vi "bmp_2_file(processed).vi"(10 "Dest":path, 11 "Image":path) -> ()   [LabVIEW 2015]
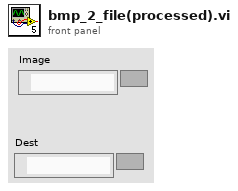
[diagram p1: front panel]
types:
  T1 = enum16{"open", "replace", "create", "open or create", "replace or create", "replace or create with confirmation"}
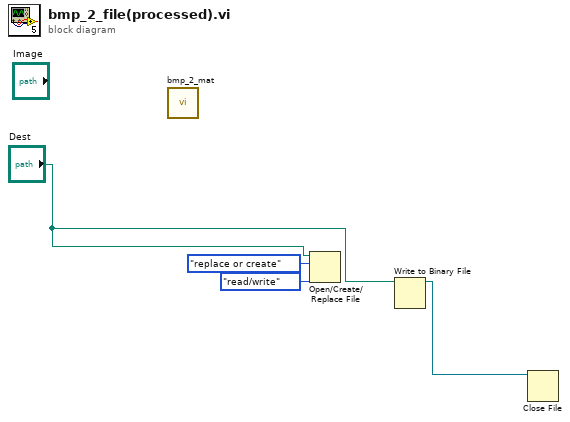
[diagram p0: block diagram]
diagram:
  n1 = call "bmp_2_mat.vi"() -> ()  [unwired: 12 in]
  n2 = Open/Create/Replace File(file path (use dialog)="Dest", operation (0:open)=T1."replace or create", access (0:read/write)=enum16{"read/write", "read-only", "write-only"}."read/write") -> ()  [unwired: 3 in, 3 out]
  n3 = Write to Binary File(file (use dialog)="Dest") -> (data=w2:cluster{}, refnum out=w1:refnum<file>)  [unwired: 4 in, 2 out]
  n4 = Close File(refnum=w1) -> ()  [unwired: 1 in, 2 out]
